vi "test_script.vi"() -> ()   [LabVIEW 2016]
uses:
  C:/Laser generated ultrasound/Labview/Kinesis Control/Thorlabs.MotionControl.Controls.dll
  Thorlabs.MotionControl.Controls.dll
  C:/Laser generated ultrasound/Labview/Kinesis Control/Thorlabs.MotionControl.KCube.BrushlessMotorCLI.dll
  Thorlabs.MotionControl.KCube.BrushlessMotorCLI.dll
panel:
  in  "step delay":u32=1500
  in  "end position":dbl=12.0
  in  "step size":dbl=0.5
  in  "stop sequence":bool
  out "GetPositionCounter":sgl
  in  "stop":bool
  in  "SerialNumber":string="28251512"
  in  "KCubeBrushlessControl":refnum<k24>(container)
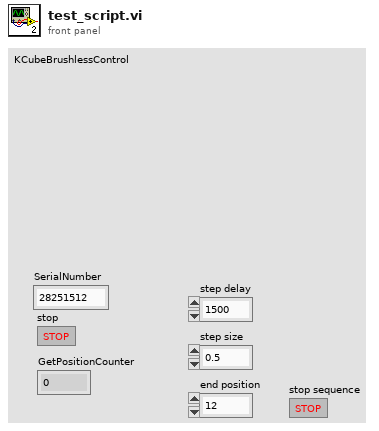
[diagram p1: front panel]
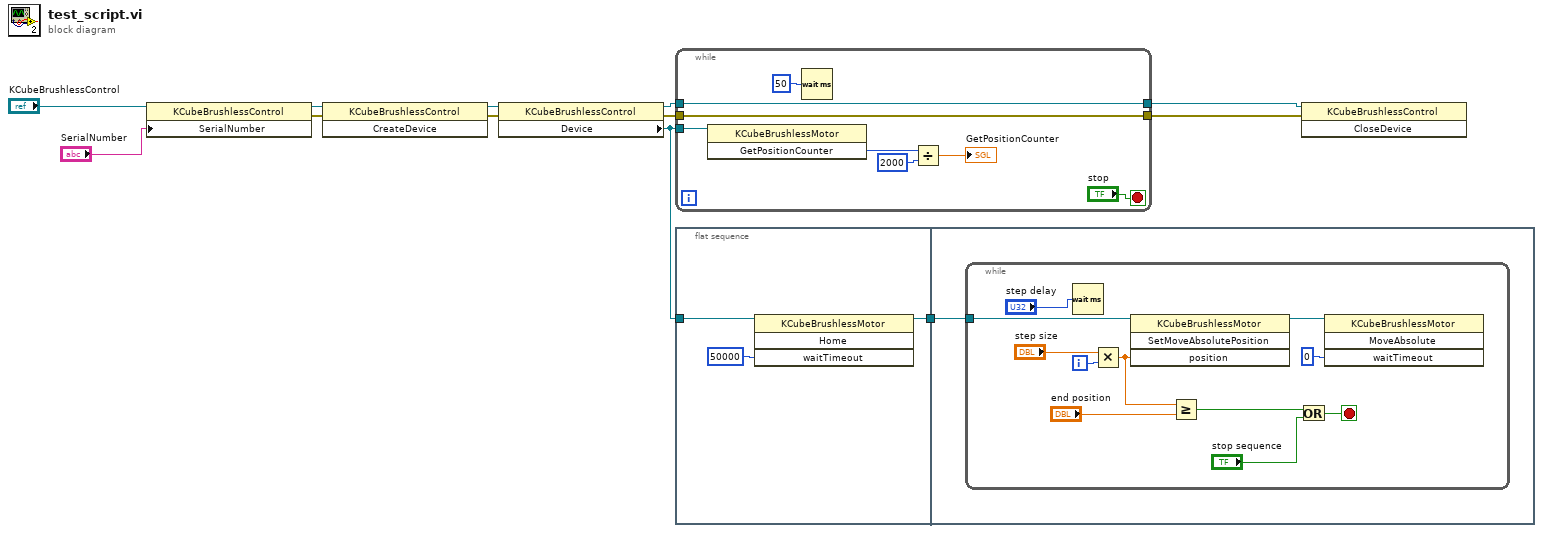
[diagram p0: block diagram]
diagram:
  n1 = property class="KCubeBrushlessControl"(reference="KCubeBrushlessControl", "SerialNumber"="SerialNumber") -> (reference out=w10:refnum<k24>, error out=w9:errorcluster)  [unwired: 1 in]
  n2 = invoke class="KCubeBrushlessControl" method="CreateDevice"(reference=w10, error in=w9) -> (reference out=w8:refnum<k24>, error out=w7:errorcluster)  [unwired: 1 in, 1 out]
  n3 = property class="KCubeBrushlessControl"(reference=w8, error in=w7) -> (reference out=w6:refnum<k24>, error out=w4:errorcluster, "Device"=w2:refnum<k24>)
  n4 = while {
    tunnel: w6 -> [w19]
    tunnel: [w19] -> w5
    tunnel: w4 -> [w18]
    tunnel: [w18] -> w3
    tunnel: w2 -> [w17]
    stop <- "stop" stop-if-true
    n5 = invoke class="KCubeBrushlessMotor" method="GetPositionCounter"(reference=w17) -> ("GetPositionCounter"=w15:i32)  [unwired: 2 in, 2 out]
    n6 = Wait (ms)(milliseconds to wait=u32 50) -> ()  [unwired: 1 out]
    n7 = Divide(x=w15, y=2000) -> (x/y=→"GetPositionCounter":dbl)
  }
  n8 = flat-sequence {
    tunnel: w2 -> [w23]
    tunnel: [w21] -> w1
    tunnel: w1 -> [w24]
    frame #0 {
      n9 = invoke class="KCubeBrushlessMotor" method="Home"(reference=w23, "waitTimeout"=50000) -> (reference out=w21:refnum<k24>)  [unwired: 2 in, 3 out]
    }
    frame #1 {
      n10 = while {
        tunnel: w24 -> [w35]
        i -> [w31]
        stop <- w26 stop-if-true
        n11 = Wait (ms)(milliseconds to wait="step delay") -> ()  [unwired: 1 out]
        n12 = Multiply(x="step size", y=w31) -> (x*y=w30:dbl)
        n13 = invoke class="KCubeBrushlessMotor" method="SetMoveAbsolutePosition"(reference=w35, "position"=w30) -> (reference out=w34:refnum<k24>)  [unwired: 2 in, 3 out]
        n14 = Greater Or Equal?(x=w30, y="end position") -> (x >= y?=w27:bool)
        n15 = Or(x=w27, y="stop sequence") -> (x .or. y?=w26:bool)
        n16 = invoke class="KCubeBrushlessMotor" method="MoveAbsolute"(reference=w34, "waitTimeout"=0) -> ()  [unwired: 2 in, 4 out]
      }
    }
  }
  n17 = invoke class="KCubeBrushlessControl" method="CloseDevice"(reference=w5, error in=w3) -> ()  [unwired: 1 in, 3 out]
